vi "Start Measurement.vi"(0 "EK-P4.lvclass":refnum<class "EK-P4.lvclass">, 11 "error in (no error)":errorcluster) -> (4 "EK-P4.lvclass 2":refnum<class "EK-P4.lvclass">, 15 "error out":errorcluster)   [LabVIEW 2016, in "EK-P4.lvclass"]
doc: "initializes connection to the Ek-P4 sensirion board using I2C"
uses:
  EK-P4.lvclass
  EK-P4.lvclass/EK-P4.ctl
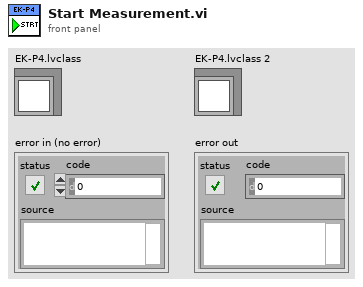
[diagram p1: front panel]
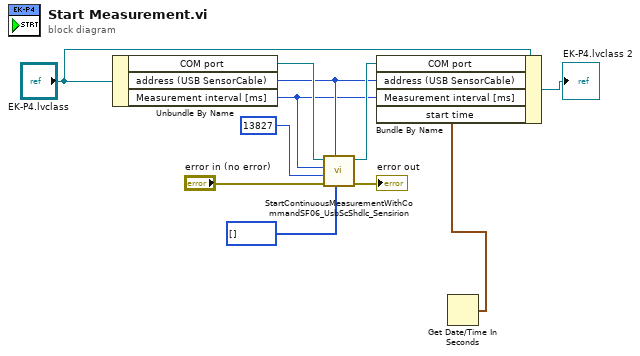
[diagram p0: block diagram]
diagram:
  n1 = Unbundle By Name("EK-P4.lvclass") -> ("COM port"=w4:refnum<visa-resource-name>, "address (USB SensorCable)"=w3:u8, "Measurement interval [ms]"=w2:u16)
  n2 = call "StartContinuousMeasurementWithCommandSF06_UsbScShdlc_Sensirion.vi"("AdditionalParameter"=u8[] [] ("AdditionalParameter\n(for used command)"), "address"=w3, "error in (no error)"="error in (no error)", "Command"=u16 13827, "Measurement interval [ms]"=w2, "COM port"=w4) -> ("error out"=→"error out":errorcluster, "COM port out"=w6:refnum<visa-resource-name>)  [unwired: 4 in]
  n3 = Get Date/Time In Seconds() -> (seconds since 1Jan1904=w1:timestamp)
  n4 = Bundle By Name(cluster="EK-P4.lvclass", "COM port"=w6, "address (USB SensorCable)"=w3, "Measurement interval [ms]"=w2, "start time"=w1) -> (→"EK-P4.lvclass 2":refnum<class "EK-P4.lvclass">)
